vi "rqcBob Create ServiceNET.vi"(8 "error in":errorcluster, 10 "port":u16, 11 "Alice's IP address":string) -> (0 "error out":errorcluster, 3 "rqcBob ServiceNET control":T1={"connection ID"=refnum, "connected?"=FALSE, "Alice's IP address"="192.168.0.92", "port"=0})   [LabVIEW 2018]
uses:
  Custom Controls/rqcBob ServiceNET control.ctl
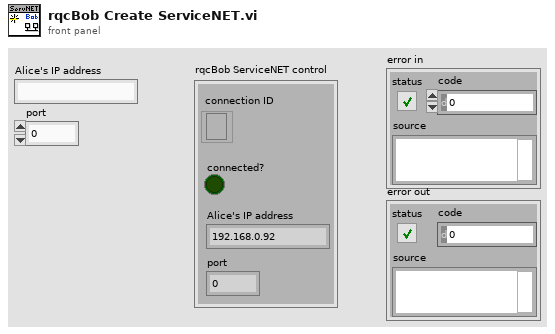
[diagram p1: front panel]
types:
  T1 = typedef "rqcBob ServiceNET control.ctl" = cluster{"connection ID":refnum<k5>, "connected?":bool, "Alice's IP address":string, "port":u16}
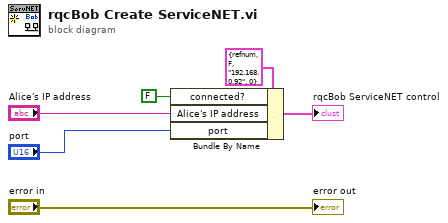
[diagram p0: block diagram]
diagram:
  n1 = Bundle By Name(cluster=T1 {"connection ID"=refnum, "connected?"=FALSE, "Alice's IP address"="192.168.0.92", "port"=0} ("rqcBob ServiceNET control"), "connected?"=FALSE, "Alice's IP address"="Alice's IP address", "port"="port") -> (→"rqcBob ServiceNET control":T1)
  "error out" <- "error in"
